vi "RegisterMat_Image.vi"(8 "error in":errorcluster, 11 "Image Reference In":T1) -> (0 "error out":errorcluster, 3 "Image Reference Out":T1, 4 "AdressOrData":u64 format="%.0x", 6 "Mat":T2)   [LabVIEW 2020, in "OpenLvVision_OpenCv.lvlib"]
doc: "Register mat for dll.\nNo malleable to breake vi inlining!"
uses:
  OpenLvVision_OpenCv.lvlib
  TypeDef/MatInfo.ctl
  TypeDef/LvDatatype.ctl
  <vilib>/OpenLvVision/OpenLvVision_Image/Management/TypeDef/OLV Image.ctl
  <vilib>/OpenLvVision/OpenLvVision_Image/DataAccess/OLV DataAccess.lvlib
  <vilib>/OpenLvVision/OpenLvVision_Image/Management/OLV Management.lvlib
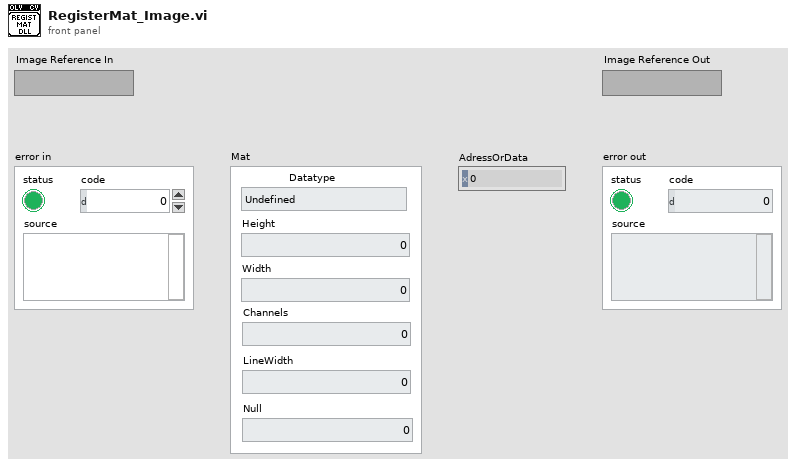
[diagram p1: front panel]
types:
  T1 = typedef "OLV OpenLvVision_Image.lvlib/OLV Management.lvlib/OLV Image.ctl" = refnum<image>
  T2 = typedef "OpenLvVision_OpenCv.lvlib/MatInfo.ctl" = cluster{"Datatype":T3, "Height":i32, "Width":i32, "Channels":i32, "LineWidth":i32, "Null":u8}
  T3 = typedef "OpenLvVision_OpenCv.lvlib/LvDatatype.ctl" = enum32{"Undefined", "U8", "I8", "U16", "I16", "U32", "I32", "U64", "I64", "SGL", "DBL", "Complex SGL", "Complex DBL", "Array 1D U8", "Array 1D I8", "Array 1D U16", "Array 1D I16", "Array 1D U32", "Array 1D I32", "Array 1D U64", "Array 1D I64", "Array 1D SGL", "Array 1D DBL", "Array 1D Complex SGL", "Array 1D Complex DBL", "Array 2D U8", "Array 2D I8", "Array 2D U16", "Array 2D I16", "Array 2D U32", "Array 2D U32_Color", "Array 2D I32", "Array 2D U64", "Array 2D U64_Color", "Array 2D I64", "Array 2D SGL", "Array 2D DBL", "Array 2D Complex SGL", "Array 2D Complex DBL", "Array 3D U8", "Array 3D I8", "Array 3D U16", "Array 3D I16", "Array 3D U32", "Array 3D I32", "Array 3D U64", "Array 3D I64", "Array 3D SGL", "Array 3D DBL", "Array 3D Complex SGL", "Array 3D Complex DBL", "Image Mono U8", "Image Mono U16", "Image Mono I16", "Image Mono SGL", "Image Color U32", "Image Color U64", "ImageComplex Sgl"}
  T4 = typedef "OLV OpenLvVision_Image.lvlib/OLV DataAccess.lvlib/OLV ImagePointer.ctl" = cluster{"ImagePointer":u64, "BorderSize":i32, "LineWidth":i32, "Width":i32, "Height":i32, "ImageFormat":T5}
  T5 = typedef "OLV OpenLvVision_Image.lvlib/OLV Management.lvlib/OLV ImageType.ctl" = enum16{"Mono U8", "Mono U16", "Mono I16", "Mono SGL", "Color U32", "Color U64", "Complex CSG"}
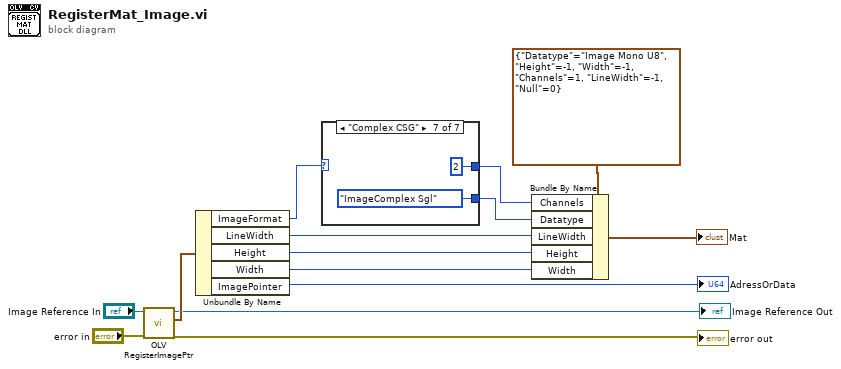
[diagram p0: block diagram]
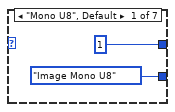
[diagram p2: hidden frame]
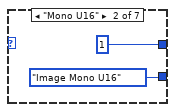
[diagram p3: hidden frame]
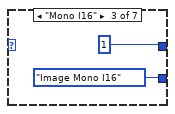
[diagram p4: hidden frame]
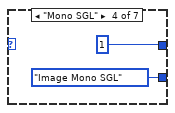
[diagram p5: hidden frame]
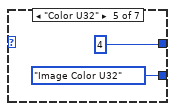
[diagram p6: hidden frame]
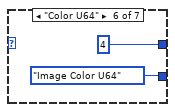
[diagram p7: hidden frame]
diagram:
  n1 = call <vilib>:"OLV RegisterImagePtr.vi"("error in"="error in", "Image Reference In"="Image Reference In") -> ("error out"=→"error out":errorcluster, "ImagePointer"=w9:T4, "Image Reference Out"=→"Image Reference Out":T1)  [unwired: 7 in]
  n2 = Unbundle By Name(w9) -> ("ImageFormat"=w1:T5, "LineWidth"=w10:i32, "Height"=w11:i32, "Width"=w12:i32, "ImagePointer"=→"AdressOrData":u64)
  n3 = case shown="\"Complex CSG\"" w1 {
    tunnel: [1 ("Channels") 1 ("Channels") 1 ("Channels") 1 ("Channels") 4 ("Channels") 4 ("Channels") 2 ("Channels")] -> w13
    tunnel: [LvDatatype."Image Mono U8" ("Datatype") LvDatatype."Image Mono U16" ("Datatype") LvDatatype."Image Mono I16" ("Datatype") LvDatatype."Image Mono SGL" ("Datatype") LvDatatype."Image Color U32" ("Datatype") LvDatatype."Image Color U64" ("Datatype") LvDatatype."ImageComplex Sgl" ("Datatype")] -> w14
    frame "Mono U8", Default {
    }
    frame "Mono U16" {
    }
    frame "Mono I16" {
    }
    frame "Mono SGL" {
    }
    frame "Color U32" {
    }
    frame "Color U64" {
    }
    frame "Complex CSG" {
    }
  }
  n4 = Bundle By Name(cluster=T2 {"Datatype"=enum."Image Mono U8", "Height"=-1, "Width"=-1, "Channels"=1, "LineWidth"=-1, "Null"=0} ("LvData"), "Channels"=w13, "Datatype"=w14, "LineWidth"=w10, "Height"=w11, "Width"=w12) -> (→"Mat":T2)
